vi "Test Histogram.vi"() -> ()   [LabVIEW 2020, in "graph_utilities.lvclass"]
uses:
  graph_utilities.lvclass
  graph_utilities.lvclass/graph_utilities.ctl
panel:
  in  "lock to bin edges":bool
  out "Histogram":cluster{"X":dbl, "Y":dbl}[](graph)
  out "Vertical Linecut":cluster{"X":dbl, "Y":dbl}[](graph)
  out "Horizontal Linecut":cluster{"X":dbl, "Y":dbl}[](graph)
  out "Intensity Graph":dbl[][](graph)
  in  "# std deviations for histogram width":dbl(slide)=1.4340101522842639 scale=0.0..5.0
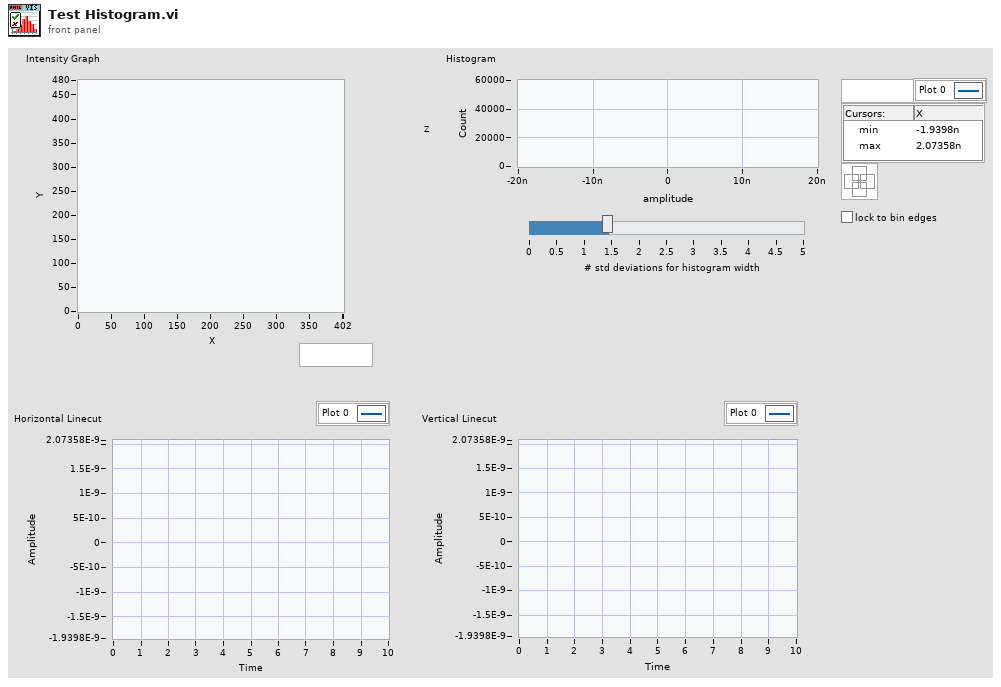
[diagram p1: front panel]
types:
  T1 = cluster{"X Values":dbl[], "Histogram: h(x)":i32[]}
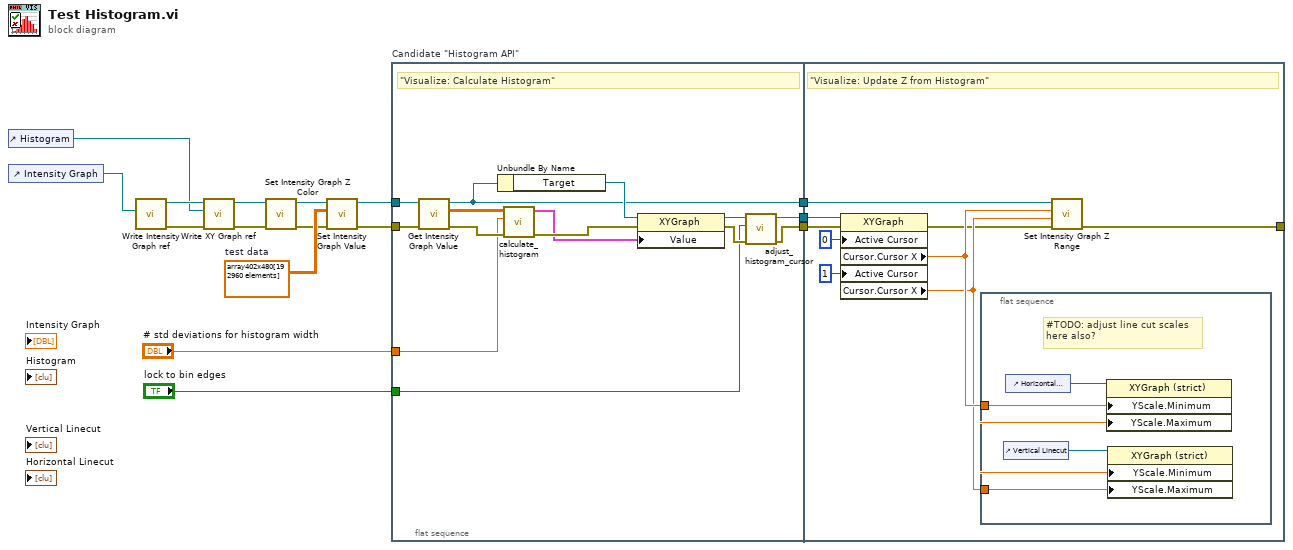
[diagram p0: block diagram]
diagram:
  w14 = dbl[][] array402x480[192960 elements]  # test data
  n1 = control-ref of="Histogram"() -> (w2:refnum<vi>)
  n2 = control-ref of="Intensity Graph"() -> (w11:refnum<vi>)
  n3 = call "Write Intensity Graph ref.vi"("Intensity Graph"=w11) -> ("error out"=w7:errorcluster, "graph_utilities out"=w6:refnum<class "graph_utilities.lvclass">)  [unwired: 9 in]
  n4 = call "Write XY Graph ref.vi"("error in (no error)"=w7, "XY Graph"=w2, "graph_utilities in"=w6) -> ("error out"=w4:errorcluster, "graph_utilities out"=w5:refnum<class "graph_utilities.lvclass">)  [unwired: 7 in]
  n5 = call "Set Intensity Graph Z Color.vi"("error in (no error)"=w4, "graph_utilities in"=w5) -> ("error out"=w13:errorcluster, "graph_utilities out"=w15:refnum<class "graph_utilities.lvclass">)  [unwired: 8 in]
  n6 = call "Set Intensity Graph Value.vi"("error in (no error)"=w13, "Value"=w14, "graph_utilities in"=w15) -> ("error out"=w12:errorcluster, "graph_utilities out"=w10:refnum<class "graph_utilities.lvclass">)  [unwired: 7 in]
  n7 = flat-sequence "Candidate \"Histogram API\"" {
    tunnel: [w30] -> w16
    tunnel: w12 -> [w26]
    tunnel: w10 -> [w27]
    tunnel: "# std deviations for histogram width" -> [w23]
    tunnel: "lock to bin edges" -> [w22]
    tunnel: [w18] -> w3
    tunnel: [w17] -> w1
    tunnel: w16 -> [w37]
    tunnel: w3 -> [w34]
    tunnel: [w32] -> _
    tunnel: w1 -> [w31]
    frame #0 {
      # "\"Visualize: Calculate Histogram\""
      n8 = call "Get Intensity Graph Value.vi"("error in (no error)"=w26, "graph_utilities in"=w27) -> ("error out"=w25:errorcluster, "Value"=w24:dbl[][], "graph_utilities out"=w18:refnum<class "graph_utilities.lvclass">)  [unwired: 7 in]
      n9 = Unbundle By Name(w18) -> ("Target"=w20:refnum<vi>)
      n10 = call "calculate_histogram.vi"("error in (no error)"=w25, "# std deviations for histogram width [1]"=w23, "2D arr Intensity Graph"=w24) -> ("error out"=w29:errorcluster, "Histogram Graph"=w21:T1)  [unwired: 5 in, 2 out]
      n11 = property class="XYGraph"(reference=w20, error in=w29, "Value"=w21) -> (reference out=w19:refnum<vi>, error out=w28:errorcluster)
      n12 = call "adjust_histogram_cursor.vi"("error in (no error)"=w28, "lock to bin edges"=w22, "histogram"=w19) -> ("error out"=w30:errorcluster, "histogram out"=w17:refnum<vi>)  [unwired: 7 in]
    }
    frame #1 {
      # "\"Visualize: Update Z from Histogram\""
      n13 = property on="Property Node" class="XYGraph"(reference=w31, error in=w37, "Active Cursor"=u32 0, "Active Cursor"=u32 1) -> (error out=w33:errorcluster, "Cursor.Cursor X"=w36:dbl, "Cursor.Cursor X"=w35:dbl)  [unwired: 1 out]
      n14 = flat-sequence {
        tunnel: w36 -> [w43]
        tunnel: w35 -> [w42]
        frame #0 {
          # "#TODO: adjust line cut scales\nhere also?"
          n15 = control-ref of="Vertical Linecut"() -> (w40:refnum<vi>)
          n16 = control-ref of="Horizontal Linecut"() -> (w41:refnum<vi>)
          n17 = property on="Property Node" class="XYGraph (strict)"(reference=w41, "YScale.Minimum"=w43, "YScale.Maximum"=w42) -> ()  [unwired: 1 in, 2 out]
          n18 = property on="Property Node" class="XYGraph (strict)"(reference=w40, "YScale.Minimum"=w43, "YScale.Maximum"=w42) -> ()  [unwired: 1 in, 2 out]
        }
      }
      n19 = call "Set Intensity Graph Z Range.vi"("error in (no error)"=w33, "Maximum [1]"=w35, "Minimum [0]"=w36, "graph_utilities in"=w34) -> ("error out"=w32:errorcluster)  [unwired: 6 in, 1 out]
    }
  }
